vi "1 sample delay 16spc.vi"(8 "input valid":bool=TRUE, 10 "delay":u8, 11 "IQ in":T1(array[cluster])=[{"I"=0.0, "Q"=0.0, "overflow"=FALSE}, {"I"=0.0, "Q"=0.0, "overflow"=FALSE}, {"I"=0.0, "Q"=0.0, "overflow"=FALSE}, {"I"=0.0, "Q"=0.0, "overflow"=FALSE}, {"I"=0.0, "Q"=0.0, "overflow"=FALSE}, {"I"=0.0, "Q"=0.0, "overflow"=FALSE}, {"I"=0.0, "Q"=0.0, "overflow"=FALSE}, {"I"=0.0, "Q"=0.0, "overflow"=FALSE}, {"I"=0.0, "Q"=0.0, "overflow"=FALSE}, {"I"=0.0, "Q"=0.0, "overflow"=FALSE}, {"I"=0.0, "Q"=0.0, "overflow"=FALSE}, {"I"=0.0, "Q"=0.0, "overflow"=FALSE}, {"I"=0.0, "Q"=0.0, "overflow"=FALSE}, {"I"=0.0, "Q"=0.0, "overflow"=FALSE}, {"I"=0.0, "Q"=0.0, "overflow"=FALSE}, {"I"=0.0, "Q"=0.0, "overflow"=FALSE}]) -> (0 "output valid":bool, 3 "IQ out":T1(array[cluster]))   [LabVIEW 2021]
doc: "sum 2 IQ datas (I+I =>I ; Q+Q =>Q ; overflow or overflow or +overflow => overflow"
types:
  T1 = cluster{"I":fxp<+/-,18,1>, "Q":fxp<+/-,18,1>, "overflow":bool}[]
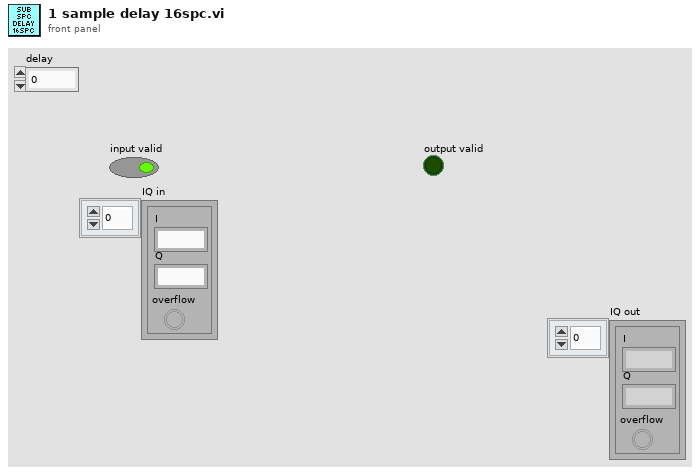
[diagram p1: front panel]
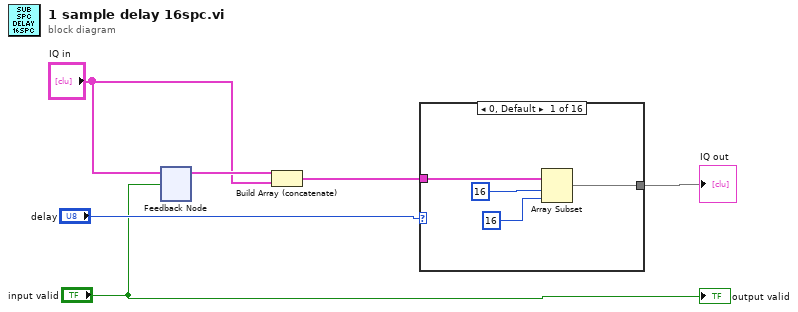
[diagram p0: block diagram]
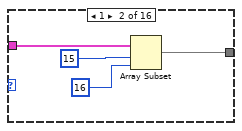
[diagram p2: hidden frame]
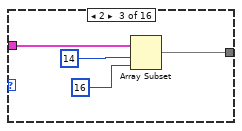
[diagram p3: hidden frame]
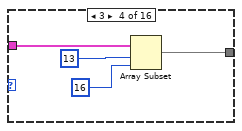
[diagram p4: hidden frame]
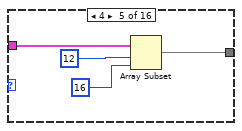
[diagram p5: hidden frame]
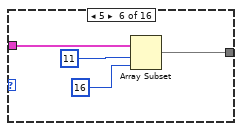
[diagram p6: hidden frame]
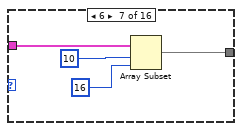
[diagram p7: hidden frame]
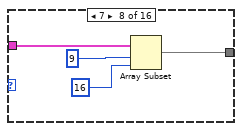
[diagram p8: hidden frame]
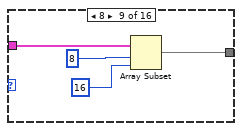
[diagram p9: hidden frame]
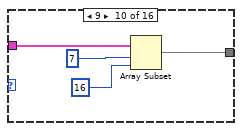
[diagram p10: hidden frame]
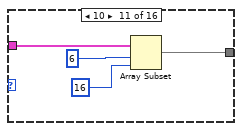
[diagram p11: hidden frame]
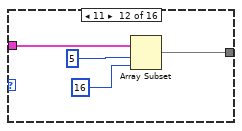
[diagram p12: hidden frame]
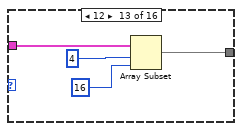
[diagram p13: hidden frame]
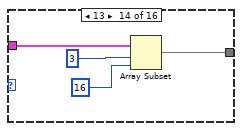
[diagram p14: hidden frame]
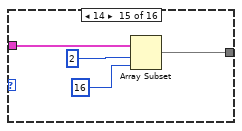
[diagram p15: hidden frame]
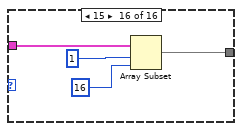
[diagram p16: hidden frame]
diagram:
  n1 = feedback #1() -> (w6:T1)  [unwired: 1 in]
  n2 = feedback-in #1("IQ in", "input valid") -> ()
  n3 = Build Array (concatenate)(w6, "IQ in") -> (w4:T1)
  n4 = case shown="0, Default" "delay" {
    tunnel: w4 -> [w10 w14 w18 w22 w26 w30 w34 w38 w42 w46 w50 w54 w58 w62 w66 w70]
    tunnel: [w8 w12 w16 w20 w24 w28 w32 w36 w40 w44 w48 w52 w56 w60 w64 w68] -> w3
    frame 0, Default {
      n5 = Array Subset(array=w10, index=16, length=16) -> (w8:T1)
    }
    frame 1 {
      n6 = Array Subset(array=w14, index=15, length=16) -> (w12:T1)
    }
    frame 2 {
      n7 = Array Subset(array=w18, index=14, length=16) -> (w16:T1)
    }
    frame 3 {
      n8 = Array Subset(array=w22, index=13, length=16) -> (w20:T1)
    }
    frame 4 {
      n9 = Array Subset(array=w26, index=12, length=16) -> (w24:T1)
    }
    frame 5 {
      n10 = Array Subset(array=w30, index=11, length=16) -> (w28:T1)
    }
    frame 6 {
      n11 = Array Subset(array=w34, index=10, length=16) -> (w32:T1)
    }
    frame 7 {
      n12 = Array Subset(array=w38, index=9, length=16) -> (w36:T1)
    }
    frame 8 {
      n13 = Array Subset(array=w42, index=8, length=16) -> (w40:T1)
    }
    frame 9 {
      n14 = Array Subset(array=w46, index=7, length=16) -> (w44:T1)
    }
    frame 10 {
      n15 = Array Subset(array=w50, index=6, length=16) -> (w48:T1)
    }
    frame 11 {
      n16 = Array Subset(array=w54, index=5, length=16) -> (w52:T1)
    }
    frame 12 {
      n17 = Array Subset(array=w58, index=4, length=16) -> (w56:T1)
    }
    frame 13 {
      n18 = Array Subset(array=w62, index=3, length=16) -> (w60:T1)
    }
    frame 14 {
      n19 = Array Subset(array=w66, index=2, length=16) -> (w64:T1)
    }
    frame 15 {
      n20 = Array Subset(array=w70, index=1, length=16) -> (w68:T1)
    }
  }
  "IQ out" <- w3
  "output valid" <- "input valid"
